vi "addJavaScriptElement.vi"(7 "Name":string, 8 "error in (no error)":errorcluster, 9 "Javascript":string, 10 "Replace? (false)":bool, 11 "tBSONDocument in":refnum<class "tBSONDocument.lvclass">) -> (0 "error out":errorcluster, 3 "tBSONDocument out":refnum<class "tBSONDocument.lvclass">)   [LabVIEW 2013, in "BSON.lvlib" / "tBSONDocument.lvclass"]
doc: "Adds Javascript to a BSON document."
uses:
  tBSONDocument.lvclass
  BSONElements/tBSONJavaScript/tBSONJavaScript.lvclass
  tBSONElement/tBSONElement.lvclass
  tBSONElement/setName.vi
  BSONElements/tBSONJavaScript/setScript.vi
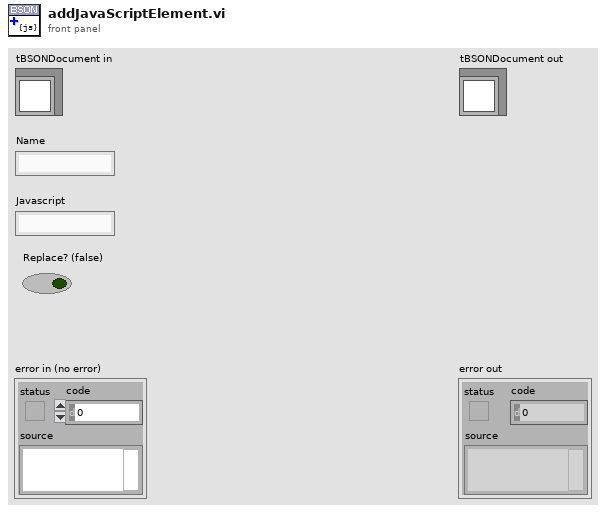
[diagram p1: front panel]
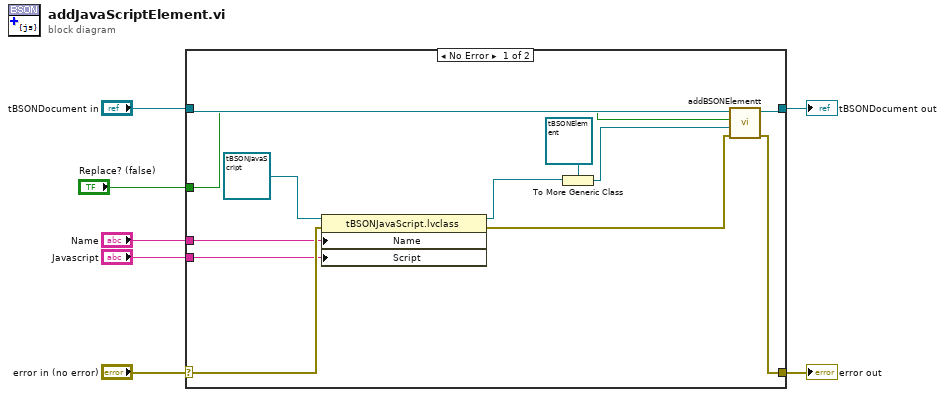
[diagram p0: block diagram]
diagram:
  n1 = case shown="No Error" "error in (no error)" {
    selector: "error in (no error)" -> [w13 w21]
    tunnel: [w14 w21] -> w6
    tunnel: [w9 w20] -> w4
    tunnel: "tBSONDocument in" -> [w16 w20]
    tunnel: "Name" -> [w11 _]
    tunnel: "Javascript" -> [w10 _]
    tunnel: "Replace? (false)" -> [w8 _]
    frame No Error {
      n2 = property class="tBSONJavaScript.lvclass"(reference=refnum<class "tBSONJavaScript.lvclass"> refnum ("BSON.lvlib:tBSONJavaScript.lvclass"), error in=w13, "Name"=w11, "Script"=w10) -> (reference out=w12:refnum<class "tBSONJavaScript.lvclass">, error out=w15:errorcluster)
      n3 = To More Generic Class(target class=refnum<class "tBSONElement.lvclass"> refnum ("BSON.lvlib:tBSONElement.lvclass"), reference=w12) -> (generic class reference=w18:refnum<class "tBSONElement.lvclass">)
      n4 = call "addBSONElementt.vi"("error in (no error)"=w15, "Element"=w18, "Replace? (false)"=w8, "tBSONDocument in"=w16) -> ("error out"=w14:errorcluster, "tBSONDocument out"=w9:refnum<class "tBSONDocument.lvclass">)  [unwired: 6 in]
    }
    frame Error {
    }
  }
  "error out" <- w6
  "tBSONDocument out" <- w4
